vi "FlatToRichnidaqmx_grpc_GetTaskAttributeStringRequest.vi"(5 "OutputClusterType":T1, 11 "InputCluster":T3) -> (3 "OutputCluster":T1)   [LabVIEW 2021, in "NI DAQmx_server.lvlib"]
uses:
  NI DAQmx_server.lvlib
  nidaqmx_grpc_GetTaskAttributeStringRequest_Flat.ctl
  nidevice_grpc_Session_Flat.ctl
  nidaqmx_grpc_TaskStringAttribute.ctl
  nidaqmx_grpc_GetTaskAttributeStringRequest.ctl
  nidevice_grpc_Session_session/nidevice_grpc_Session_session.lvclass
  nidaqmx_grpc_GetTaskAttributeStringRequest_attribute_enum/nidaqmx_grpc_GetTaskAttributeStringRequest_attribute_enum.lvclass
  nidevice_grpc_Session.ctl
  nidevice_grpc_Session_session/nidevice_grpc_Session_session.lvclass/nidevice_grpc_Session_session.ctl
  nidaqmx_grpc_GetTaskAttributeStringRequest_attribute_enum/nidaqmx_grpc_GetTaskAttributeStringRequest_attribute_enum.lvclass/nidaqmx_grpc_GetTaskAttributeStringRequest_attribute_enum.ctl
  nidevice_grpc_Session_session/Setname.vi
  nidevice_grpc_Session_session/Setid.vi
  nidevice_grpc_Session_session/GetFieldFromProtobufIndexnidevice_grpc_Session_session.vi
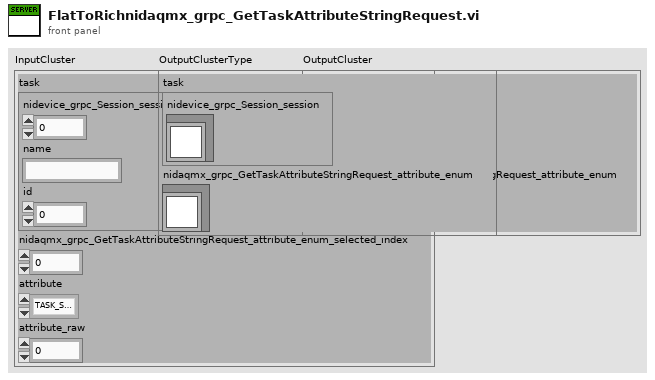
[diagram p1: front panel]
types:
  T1 = typedef "NI DAQmx_server.lvlib/nidaqmx_grpc_GetTaskAttributeStringRequest.ctl" = cluster{"task":T2, "nidaqmx_grpc_GetTaskAttributeStringRequest_attribute_enum":refnum<class "nidaqmx_grpc_GetTaskAttributeStringRequest_attribute_enum.lvclass">}
  T2 = typedef "NI DAQmx_server.lvlib/nidevice_grpc_Session.ctl" = cluster{"nidevice_grpc_Session_session":refnum<class "nidevice_grpc_Session_session.lvclass">}
  T3 = typedef "NI DAQmx_server.lvlib/nidaqmx_grpc_GetTaskAttributeStringRequest_Flat.ctl" = cluster{"task":T4, "nidaqmx_grpc_GetTaskAttributeStringRequest_attribute_enum_selected_index":i32, "attribute":T5, "attribute_raw":i32}
  T4 = typedef "NI DAQmx_server.lvlib/nidevice_grpc_Session_Flat.ctl" = cluster{"nidevice_grpc_Session_session_selected_index":i32, "name":string, "id":u32}
  T5 = typedef "NI DAQmx_server.lvlib/nidaqmx_grpc_TaskStringAttribute.ctl" = enum32{"TASK_STRING_ATTRIBUTE_UNSPECIFIED", "TASK_ATTRIBUTE_CHANNELS", "TASK_ATTRIBUTE_NAME", "TASK_ATTRIBUTE_DEVICES"}
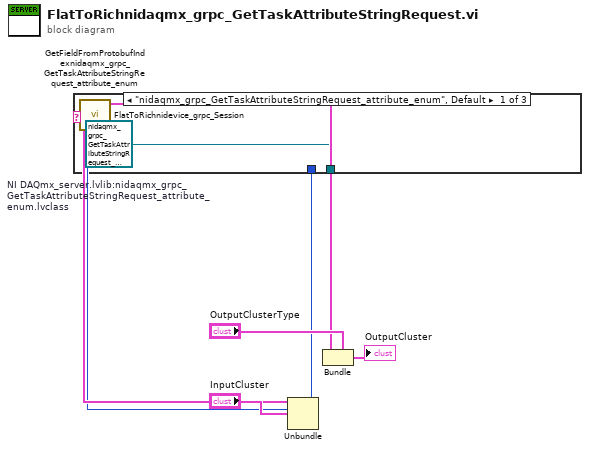
[diagram p0: block diagram]
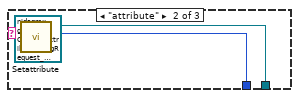
[diagram p2: hidden frame]
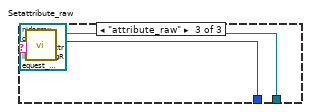
[diagram p3: hidden frame]
diagram:
  n1 = Unbundle "Unbundle"("InputCluster") -> ("task"=w7:T4, "nidaqmx_grpc_GetTaskAttributeStringRequest_attribute_enum_selected_index"=w5:i32, "attribute"=w2:T5, "attribute_raw"=w1:i32)
  n2 = call "GetFieldFromProtobufIndexnidaqmx_grpc_GetTaskAttributeStringRequest_attribute_enum.vi"("protobuf index"=w5) -> ("oneof field name"=w4:string)
  n3 = case "nidaqmx_grpc_GetTaskAttributeStringRequest_attribute_enum" shown="\"nidaqmx_grpc_GetTaskAttributeStringRequest_attribute_enum\", Default" w4 {
    tunnel: [w11 w13 w16] -> w3
    tunnel: w2 -> [_ w14 _]
    tunnel: w1 -> [_ _ w17]
    frame "nidaqmx_grpc_GetTaskAttributeStringRequest_attribute_enum", Default {
      w11 = refnum<class "nidaqmx_grpc_GetTaskAttributeStringRequest_attribute_enum.lvclass"> refnum  # NI DAQmx_server.lvlib:nidaqmx_grpc_GetTaskAttributeStringRequest_attribute_enum.lvclass
    }
    frame "attribute" {
      n4 = call "Setattribute.vi"("Set_Val"=w14, "OneOfTemplate in"=refnum<class "nidaqmx_grpc_GetTaskAttributeStringRequest_attribute_enum.lvclass"> refnum) -> ("OneOfTemplate out"=w13:refnum<class "nidaqmx_grpc_GetTaskAttributeStringRequest_attribute_enum.lvclass">)  [unwired: 8 in, 1 out]
    }
    frame "attribute_raw" {
      n5 = call "Setattribute_raw.vi"("Set_Val"=w17, "OneOfTemplate in"=refnum<class "nidaqmx_grpc_GetTaskAttributeStringRequest_attribute_enum.lvclass"> refnum) -> ("OneOfTemplate out"=w16:refnum<class "nidaqmx_grpc_GetTaskAttributeStringRequest_attribute_enum.lvclass">)  [unwired: 8 in, 1 out]
    }
  }
  n6 = call "FlatToRichnidevice_grpc_Session.vi"("InputCluster"=w7) -> ("OutputCluster"=w6:T2)  [unwired: 10 in]
  n7 = Bundle "Bundle"(cluster="OutputClusterType", "task"=w6, "nidaqmx_grpc_GetTaskAttributeStringRequest_attribute_enum"=w3) -> (→"OutputCluster":T1)
